vi "Odometria3.vi"(6 "left motor ccw velocity (rad/s)":dbl, 9 "Arrastrado":dbl[](array[numeric]), 10 "Zigma":dbl[](array[numeric]), 11 "right motor ccw velocity (rad/s)":dbl) -> (2 "Posicion estimada":ext[](array[numeric]), 3 "Velocidad actual":dbl[](array[numeric]))   [LabVIEW 2011]
uses:
  <vilib>/Analysis/Matrix/Datatypes/RealMatrix.ctl
  <vilib>/Analysis/_algsub.llb/Real PseudoInverse Matrix.vi
  <vilib>/Analysis/baseanly.llb/A x Vector.vi
  <vilib>/Analysis/Matrix/Numeric/Conversions/Array To Matrix - RA.vi
  <vilib>/Analysis/baseanly.llb/Real Inverse Matrix.vi
  <vilib>/Analysis/baseanly.llb/Real A x B.vi
  <vilib>/Analysis/NI_AALPro.lvlib
  <vilib>/Analysis/NI_AALBase.lvlib
  <vilib>/Analysis/Matrix/NI_Matrix.lvlib
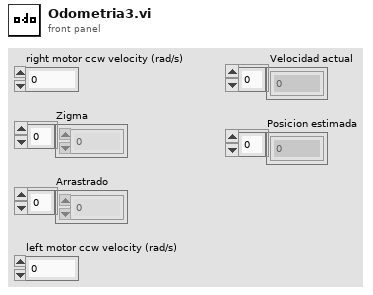
[diagram p1: front panel]
types:
  T1 = typedef "NI_Matrix.lvlib/RealMatrix.ctl" = dbl[][]
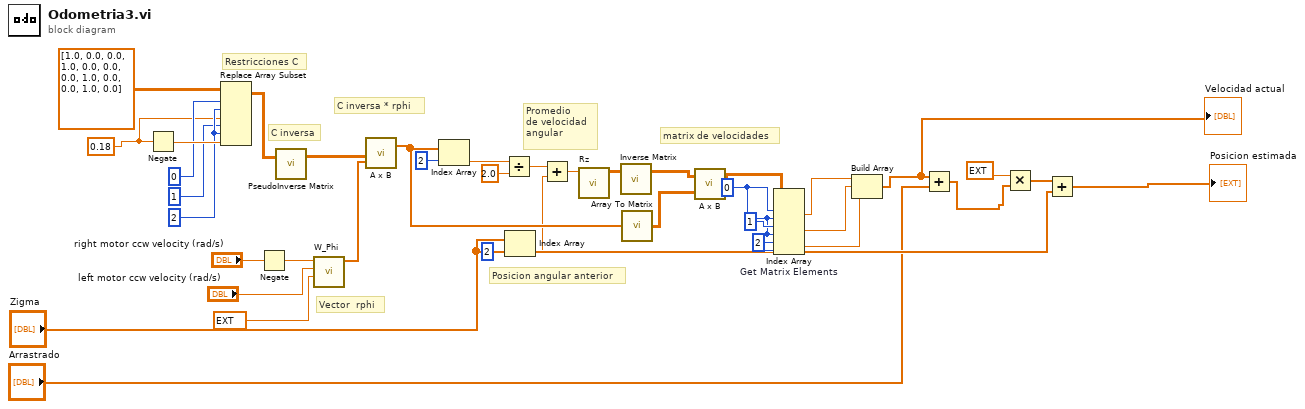
[diagram p0: block diagram]
diagram:
  w7 = 0.18
  w11 = 2
  w32 = 0 ("index (row)")
  # "matrix de velocidades"
  # "Promedio \nde velocidad \nangular"
  # "C inversa * rphi"
  # "C inversa"
  # "Vector  rphi"
  # "Posicion angular anterior"
  # "Restricciones C"
  n1 = Negate(x=w7) -> (-x=w12:dbl)
  n2 = Replace Array Subset(array=T1 [[1.0, 0.0, 0.0], [1.0, 0.0, 0.0], [0.0, 1.0, 0.0], [0.0, 1.0, 0.0]] ("Real Matrix"), new element #1=w7, index (row) #1=0, index (col) #1=w11, new element #2=w12, index (row) #2=1, index (col) #2=w11) -> (w8:T1)
  n3 = Negate(x="right motor ccw velocity (rad/s)") -> (-x=w17:dbl)
  n4 = call-poly <vilib>:"PseudoInverse Matrix.vi"("Input Matrix"=w8) -> ("PseudoInverse Matrix"=w19:T1)  [unwired: 1 in, 1 out]
  n5 = call "W_Phi.vi"("Radio"=ext 0.025 ("Numeric"), "left motor ccw velocity (rad/s)"="left motor ccw velocity (rad/s)", "right motor ccw velocity (rad/s)"=w17) -> ("Array out"=w20:ext[])  [unwired: 8 in]
  n6 = call-poly <vilib>:"A x B.vi"("Vector"=w20, "A"=w19) -> ("A x Vector"=w30:dbl[])  [unwired: 1 out]
  n7 = Index Array(array=w30, index=2) -> (element=w23:dbl)
  n8 = Divide(x=w23, y=2.0) -> (x/y=w25:dbl)
  n9 = Index Array(array="Zigma", index=2) -> (element=w26:dbl)
  n10 = Add(x=w25, y=w26) -> (x+y=w27:dbl)
  n11 = call "Rz.vi"("theta"=w27) -> ("RotacionalZ"=w28:T1)  [unwired: 10 in]
  n12 = call-poly <vilib>:"Inverse Matrix.vi"("Input Matrix"=w28) -> ("Inverse Matrix"=w5:T1)  [unwired: 1 in, 1 out]
  n13 = call-poly <vilib>:"Array To Matrix.vi"("Real 1D Array"=w30) -> ("Real Matrix (Column Vector)"=w6:T1)
  n14 = call-poly <vilib>:"A x B.vi"("B"=w6, "A"=w5) -> ("A x B"=w4:T1)  [unwired: 1 out]
  n15 = Index Array "Get Matrix Elements"(array=w4, index (row) #1=w32, index (col) #1=w32, index (row) #2=1 ("index (row)"), index (col) #2=w32, index (row) #3=2 ("index (row)"), index (col) #3=w32) -> (element #1=w31:dbl, element #2=w35:dbl, element #3=w36:dbl)
  n16 = Build Array(w31, w35, w36) -> (w37:dbl[])
  "Velocidad actual" <- w37
  n17 = Add(x=w37, y="Arrastrado") -> (x+y=w2:dbl[])
  n18 = Multiply(x=ext 0.01 ("Numeric"), y=w2) -> (x*y=w3:ext[])
  n19 = Add(x=w3, y="Zigma") -> (x+y=→"Posicion estimada":ext[])
